vi "TriggerRotationPostAcquire.vi"(0 "Microscope in":refnum<class "Microscope.lvclass">, 11 "error in (no error)":errorcluster) -> (4 "Microscope out":refnum<class "Microscope.lvclass">, 15 "error out":errorcluster)   [LabVIEW 2012, in "Microscope.lvclass"]
uses:
  classes/Microscope.lvclass
  classes/Microscope.lvclass/Microscope.ctl
  variables/GlobalUI.vi
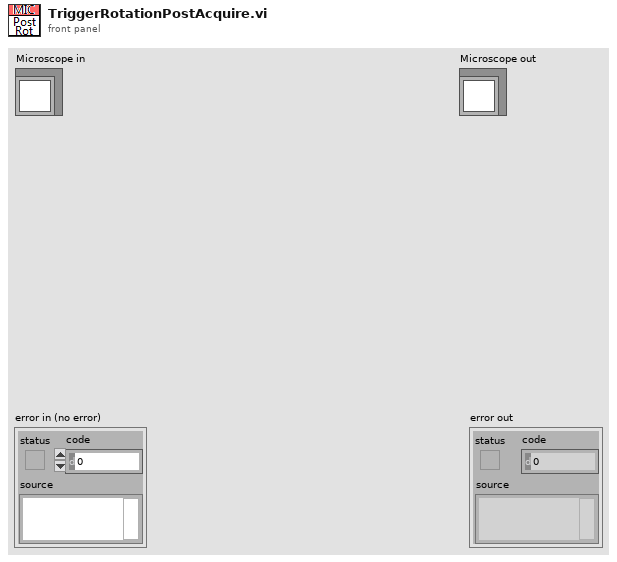
[diagram p1: front panel]
types:
  T1 = typedef "ScanMode.ctl" = enum16{"None", "Continuous", "Point Scan (CH3 cursor)", "Point Scan Move (CH3 cursor)", "Grab", "Grab Move Stage", "Grab Move Z-stage", "Cont. Move Z-stage", "Spec Move Stage", "Spec Move Cont", "Surf Calib"}
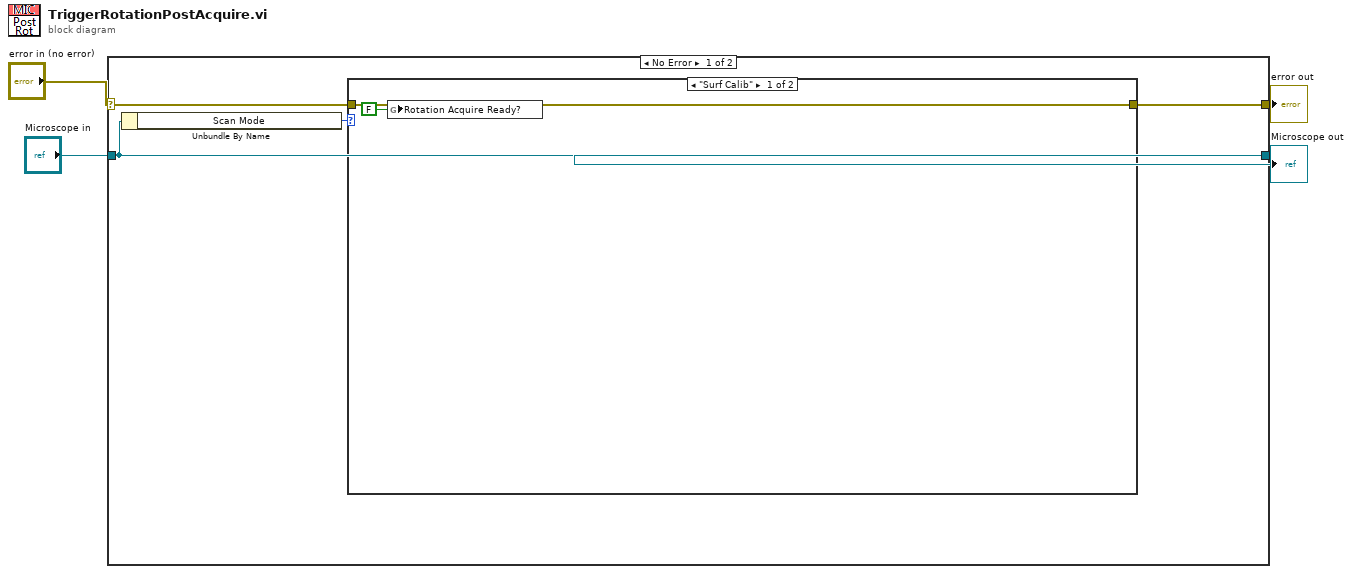
[diagram p0: block diagram]
diagram:
  n1 = case shown="No Error" "error in (no error)" {
    selector: "error in (no error)" -> [w7 w13]
    tunnel: [w6 w13] -> w3
    tunnel: [w8 w12] -> w1
    tunnel: "Microscope in" -> [w8 w12]
    frame No Error {
      n2 = Unbundle By Name(w8) -> ("Scan Mode"=w5:T1)
      n3 = case shown="\"Surf Calib\"" w5 {
        tunnel: w7 -> [w9 w11]
        tunnel: [w9 w11] -> w6
        frame "Surf Calib" {
          n4 = global write "GlobalUI.vi" "Rotation Acquire Ready?"(FALSE ("Rotation Acquire Ready?")) -> ()
        }
        frame "None", Default {
        }
      }
    }
    frame Error {
    }
  }
  "error out" <- w3
  "Microscope out" <- w1
